vi "Send Configure StartVelocity.vi"(7 "Message Priority (Normal)":T1=enum."Normal", 8 "error in (no error)":errorcluster, 9 "StartVelocity":dbl, 10 "AxisNumber":u8, 11 "Message Enqueuer":refnum<class "Message Enqueuer.lvclass">) -> (0 "error out":errorcluster, 3 "Message Enqueuer out":refnum<class "Message Enqueuer.lvclass">)   [LabVIEW 2015, in "CS++Motor.lvlib" / "Configure StartVelocity Msg.lvclass"]
doc: "Sends the <B>CS++Motor.lvlib:Configure StartVelocity Msg.lvclass</B> message.\n\n<B>CS++Motor.lvlib:CS++Motor.lvclass:Configure StartVelocity.vi</B> Description:\n\nConfigures the start (minimum) velocity of the axis."
uses:
  Configure StartVelocity Msg.lvclass
  <vilib>/ActorFramework/Message Enqueuer/Message Enqueuer.lvclass
  <vilib>/ActorFramework/Message Enqueuer/Message Priority.ctl
  Configure StartVelocity Msg.lvclass/Configure StartVelocity Msg.ctl
  <vilib>/ActorFramework/Message Enqueuer/Message Enqueuer.lvclass/Message Enqueuer.ctl
  <vilib>/ActorFramework/Message Priority Queue/Priority Enqueue.vi
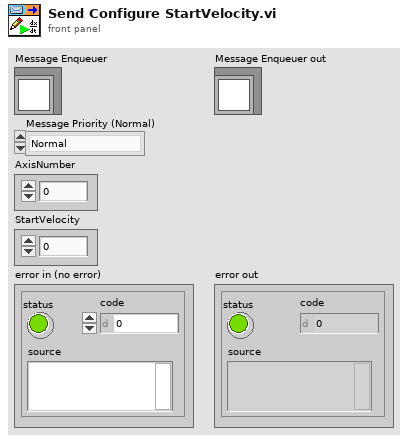
[diagram p1: front panel]
types:
  T1 = typedef "Actor Framework.lvlib/Message Enqueuer.lvclass/Message Priority.ctl" = enum16{"Low", "Normal", "High"}
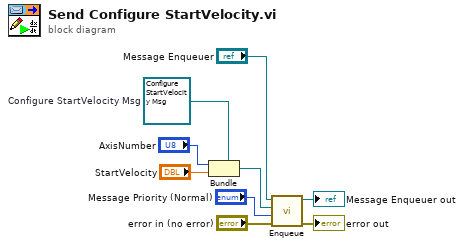
[diagram p0: block diagram]
diagram:
  w3 = refnum<class "Configure StartVelocity Msg.lvclass"> refnum  # Configure StartVelocity Msg
  n1 = Bundle(cluster=w3, "AxisNumber", "StartVelocity") -> (w6:refnum<class "Configure StartVelocity Msg.lvclass">)
  n2 = call <vilib>:"Enqueue.vi"("error in (no error)"="error in (no error)", "Message Priority (Normal)"="Message Priority (Normal)", "Message"=w6, "Message Enqueuer in"="Message Enqueuer") -> ("error out"=→"error out":errorcluster, "Message Enqueuer out"=→"Message Enqueuer out":refnum<class "Message Enqueuer.lvclass">)  [unwired: 6 in]
